vi "serverstreaming_client.vi"() -> ()   [LabVIEW 2019]
uses:
  Generated_client/RPC Messages/Request.ctl
  Generated_client/RPC Messages/Request_request_oneof/Request_request_oneof.lvclass
  Generated_client/RPC Messages/Request_request_oneof/Request_request_oneof.lvclass/Request_request_oneof.ctl
  Generated_client/RPC Messages/Response_response_oneof/Response_response_oneof.lvclass/Response_response_oneof.ctl
  Generated_client/Generated_client.lvlib
  Generated_client/RPC Messages/Response_response_oneof/Response_response_oneof.lvclass
panel:
  out "error out":errorcluster
  out "results":string[](array[string])
  out "resp_id":i32[](array[numeric])
  out "new_age":i32[](array[numeric])
  in  "age":i32
  in  "req_id":i32
  in  "message":string
  in  "req_oneof":enum16{"message", "req_id"}(ring)
  in  "error in":errorcluster
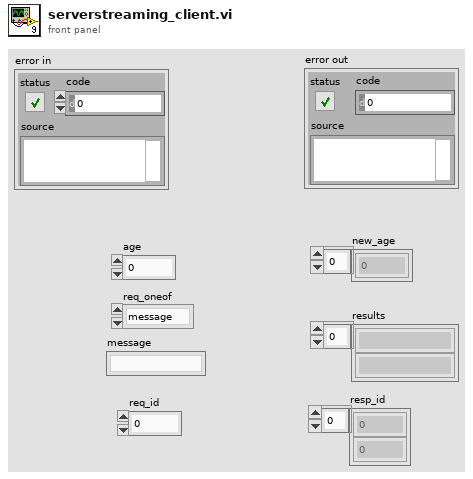
[diagram p1: front panel]
types:
  T1 = typedef "Generated_client.lvlib/Request.ctl" = cluster{"age":i32, "Request_request_oneof":refnum<class "Request_request_oneof.lvclass">}
  T2 = typedef "grpc-lvsupport-release.lvlib/grpcId.ctl" = u64
  T3 = typedef "Generated_client.lvlib/Response.ctl" = cluster{"new_age":i32, "Response_response_oneof":refnum<class "Response_response_oneof.lvclass">}
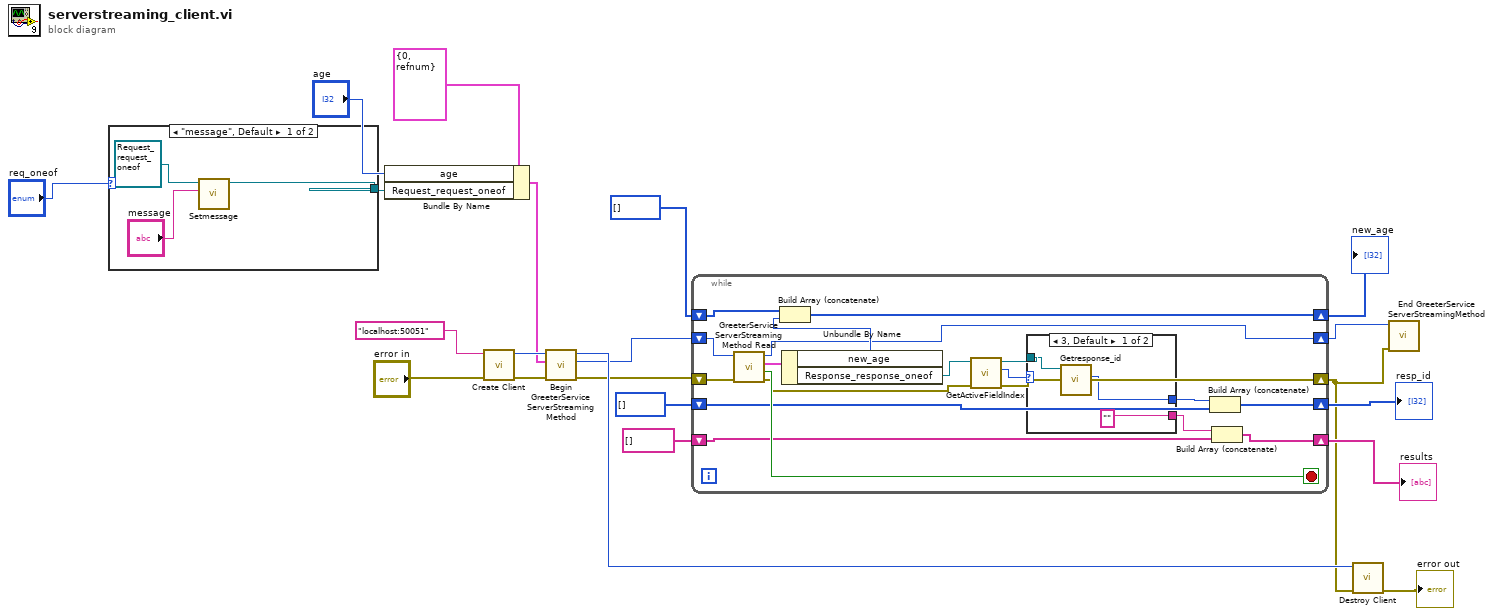
[diagram p0: block diagram]
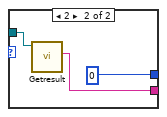
[diagram p2: hidden frame]
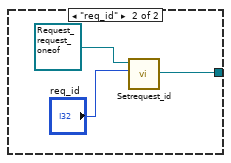
[diagram p3: hidden frame]
diagram:
  n1 = case shown="\"message\", Default" "req_oneof" {
    tunnel: [w22 w25] -> w17
    frame "message", Default {
      n2 = call "Setmessage.vi"("Set_Val"="message", "OneOfTemplate in"=refnum<class "Request_request_oneof.lvclass"> refnum) -> ("OneOfTemplate out"=w22:refnum<class "Request_request_oneof.lvclass">)  [unwired: 8 in, 1 out]
    }
    frame "req_id" {
      n3 = call "Setrequest_id.vi"("Set_Val"="req_id", "OneOfTemplate in"=refnum<class "Request_request_oneof.lvclass"> refnum) -> ("OneOfTemplate out"=w25:refnum<class "Request_request_oneof.lvclass">)  [unwired: 8 in, 1 out]
    }
  }
  n4 = Bundle By Name(cluster=T1 {"age"=0, "Request_request_oneof"=refnum} ("Request"), "age"="age", "Request_request_oneof"=w17) -> (w13:T1)
  n5 = call "Create Client.vi"("error in"="error in", "address"="localhost:50051") -> ("error out"=w14:errorcluster, "gRPC ID Out"=w15:T2)  [unwired: 8 in]
  n6 = call "Begin GreeterService ServerStreamingMethod.vi"("error in"=w14, "Request Data"=w13, "gRPC ID"=w15) -> ("error out"=w11:errorcluster, "Call Id Out"=w3:T2, "gRPC ID out"=w12:T2)  [unwired: 6 in]
  n7 = while {
    shift-right: [w30] -> w1
    shift-left: w11 -> [w46]
    shift-right: [w42] -> w7
    shift-left: i32[] [] -> [w43]
    shift-right: [w35] -> w5
    shift-left: string[] [] -> [w36]
    shift-right: [w32] -> w6
    shift-left: i32[] [] -> [w33]
    shift-right: [w28] -> w2
    shift-left: w3 -> [w29]
    stop <- w38 stop-if-true
    n8 = call "GreeterService ServerStreamingMethod Read.vi"("error in"=w46, "Call ID in"=w29) -> ("error out"=w31:errorcluster, "Success"=w38:bool, "Response Data"=w45:T3, "Call ID"=w28:T2)  [unwired: 6 in]
    n9 = Unbundle By Name(w45) -> ("new_age"=w44:i32, "Response_response_oneof"=w41:refnum<class "Response_response_oneof.lvclass">)
    n10 = Build Array (concatenate)(w43, w44) -> (w42:i32[])
    n11 = call "GetActiveFieldIndex.vi"("error in (no error)"=w31, "OneOfTemplate in"=w41) -> ("error out"=w30:errorcluster, "Active Field Index"=w40:i32, "OneOfTemplate out"=w39:refnum<class "Response_response_oneof.lvclass">)  [unwired: 7 in]
    n12 = case shown="3, Default" w40 {
      tunnel: w39 -> [w49 w52]
      tunnel: ["" ("Get_Val") w51] -> w37
      tunnel: [w48 0 ("Get_Val")] -> w34
      frame 3, Default {
        n13 = call "Getresponse_id.vi"("OneOfTemplate in"=w49) -> ("Get_Val"=w48:i32)  [unwired: 8 in, 2 out]
      }
      frame 2 {
        n14 = call "Getresult.vi"("OneOfTemplate in"=w52) -> ("Get_Val"=w51:string)  [unwired: 8 in, 2 out]
      }
    }
    n15 = Build Array (concatenate)(w34, w33) -> (w32:i32[])
    n16 = Build Array (concatenate)(w37, w36) -> (w35:string[])
  }
  "new_age" <- w7
  "resp_id" <- w6
  "results" <- w5
  n17 = call "Destroy Client.vi"("error in"=w1, "gRPC ID"=w12) -> ("error out"=→"error out":errorcluster)  [unwired: 9 in]
  n18 = call "End GreeterService ServerStreamingMethod.vi"("error in"=w1, "Call ID in"=w2) -> ()  [unwired: 8 in, 2 out]
